vi "Build Async.vi"(10 "Build":bool[](array[boolean]), 11 "Builder in":refnum<class "Builder.lvclass">) -> ()   [LabVIEW 2020, in "Builder Tools.lvlib" / "Builder.lvclass"]
uses:
  Builder.lvclass
  Builder.lvclass/Builder.ctl
  Build/Build.lvclass
  Build Events API/Build Events API.lvclass
  Builder Core/Builder Core.lvlib
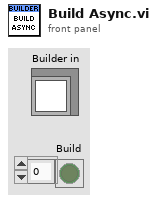
[diagram p1: front panel]
types:
  T1 = typedef "Builder Core.lvlib/Version.ctl" = cluster{"Major":u16, "Minor":u16, "Fix":u16, "Build":u16}
  T2 = typedef "Builder Tools.lvlib/Builder.lvclass/Build Step.ctl" = cluster{"Info":T3, "Build":refnum<class "Build.lvclass">}
  T3 = typedef "Builder Tools.lvlib/Build Info.ctl" = cluster{"Project Path":path, "Target":string, "Build Spec":string}
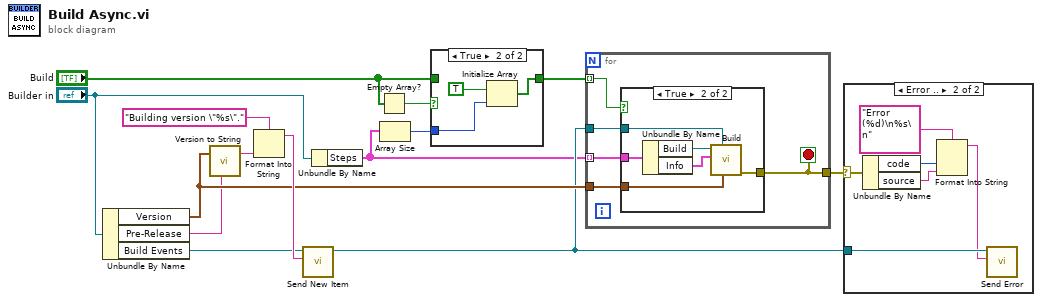
[diagram p0: block diagram]
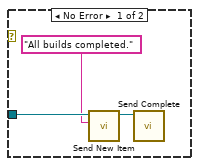
[diagram p3: hidden frame]
diagram:
  n1 = Unbundle By Name("Builder in") -> ("Version"=w9:T1, "Pre-Release"=w8:string, "Build Events"=w11:refnum<class "Build Events API.lvclass">)
  n2 = call "Version to String.vi"("Version"=w9, "Pre-Release (None)"=w8) -> ("Version String"=w13:string)  [unwired: 5 in]
  n3 = Format Into String(format string="Building version \"%s\".", w13) -> (resulting string=w12:string)  [unwired: 2 in, 1 out]
  n4 = call "Send New Item.vi"("Message"=w12, "Build Events API in"=w11) -> ("Build Events API out"=w7:refnum<class "Build Events API.lvclass">)  [unwired: 8 in, 1 out]
  n5 = Unbundle By Name("Builder in") -> ("Steps"=w5:T2[])
  n6 = Empty Array?(array="Build") -> (empty?=w4:bool)
  n7 = Array Size(array=w5) -> (size(s)=w3:i32)
  n8 = case shown="True" w4 {
    tunnel: w3 -> [_ w17]
    tunnel: "Build" -> [w15 _]
    tunnel: [w15 w16] -> w1
    frame False {
    }
    frame True {
      n9 = Initialize Array(TRUE, w17) -> (w16:bool[])
    }
  }
  n10 = for {
    tunnel: w5 -> [w23] mode=indexing
    tunnel: w7 -> [w22]
    tunnel: w9 -> [w21]
    tunnel: [w20] -> w6
    tunnel: w1 -> [w19] mode=indexing
    stop <- w20 stop-if-true
    n11 = case shown="True" w19 {
      tunnel: w23 -> [_ w29]
      tunnel: w22 -> [_ w27]
      tunnel: w21 -> [_ w25]
      tunnel: [_ w24] -> w20
      frame False {
      }
      frame True {
        n12 = Unbundle By Name(w29) -> ("Build"=w28:refnum<class "Build.lvclass">, "Info"=w26:T3)
        n13 = call-dynamic "Build.vi"("Version"=w25, "Build Events"=w27, "Build Info"=w26, "Build in"=w28) -> ("error out"=w24:errorcluster)  [unwired: 7 in]
      }
    }
  }
  n14 = case shown="Error .." w6 {
    selector: w6 -> [_ w38]
    tunnel: w7 -> [w32 w34]
    frame No Error {
      n15 = call "Send New Item.vi"("Message"="All builds completed.", "Build Events API in"=w32) -> ("Build Events API out"=w31:refnum<class "Build Events API.lvclass">)  [unwired: 8 in, 1 out]
      n16 = call "Send Complete.vi"("Build Events API in"=w31) -> ()  [unwired: 9 in, 2 out]
    }
    frame Error {
      n17 = Unbundle By Name(w38) -> ("code"=w37:i32, "source"=w35:string)
      n18 = Format Into String(format string="Error (%d)\n%s\n", w37, w35) -> (resulting string=w33:string)  [unwired: 2 in, 1 out]
      n19 = call "Send Error.vi"("Message"=w33, "Build Events API in"=w34) -> ()  [unwired: 8 in, 2 out]
    }
  }
